vi "Variant to config data - Read.vi"(7 "Section Name":string, 8 "error in (no error)":errorcluster, 9 "Control in":refnum<vi>, 10 "Key Name":string, 11 "FIle refnum IN":T1) -> (0 "error out":errorcluster, 2 "Value":variant, 3 "Refnum out":T1)   [LabVIEW 2017]
uses:
  <vilib>/Utility/config.llb/Config Data RefNum.ctl
  <vilib>/Utility/config.llb/Read Key (String).vi
  <vilib>/Utility/config.llb/Read Key (Double).vi
  <vilib>/Utility/config.llb/Read Key (Boolean).vi
  <vilib>/Utility/config.llb/Read Key (I32).vi
  <vilib>/Utility/config.llb/Read Key (U32).vi
  <vilib>/Utility/config.llb/NI_LVConfig.lvlib
  <vilib>/Utility/Data Type/NI_Data Type.lvlib
panel:
  out "found?":bool
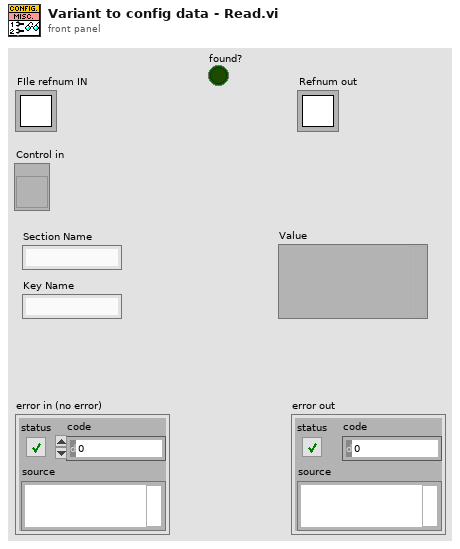
[diagram p1: front panel]
types:
  T1 = typedef "NI_LVConfig.lvlib/Config Data RefNum.ctl" = refnum<k1>
  T2 = typedef "NI_Data Type.lvlib/Data Type.ctl" = enum8{"Invalid Type", "Void", "I8", "I16", "I32", "I64", "U8", "U16", "U32", "U64", "Single Float", "Double Float", "Extended Float", "Single Complex", "Double Complex", "Extended Complex", "Enum U8", "Enum U16", "Enum U32", "Enum U64", "Single Float With Unit", "Double Float With Unit", "Extended Float With Unit", "Single Complex with Unit", "Double Complex with Unit", "Extended Complex with Unit", "Boolean", "String", "Path", "Picture", "Tag", "Array", "Cluster", "Variant", "LV Variant", "Waveform", "Timestamp", "Digital Waveform", "Digital Data", "ExpressData", "Refnum", "External Data", "VI", "Poly VI", "LabVIEW Class Instance", "Fixed Point"}
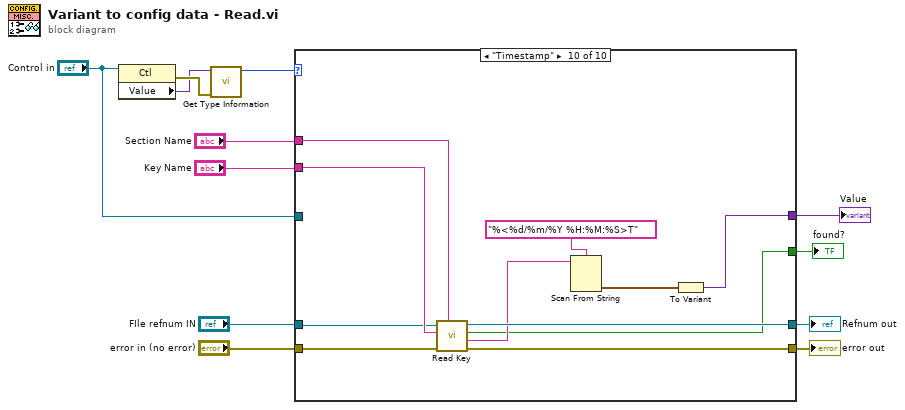
[diagram p0: block diagram]
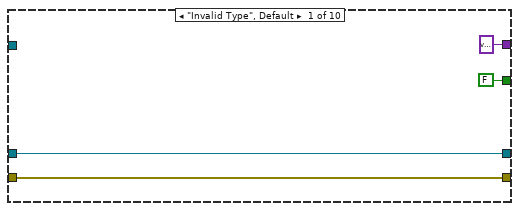
[diagram p2: hidden frame]
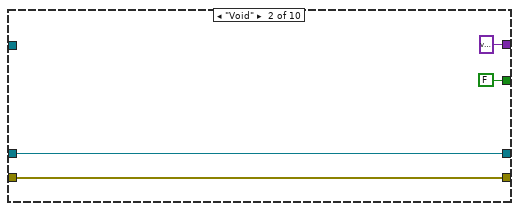
[diagram p3: hidden frame]
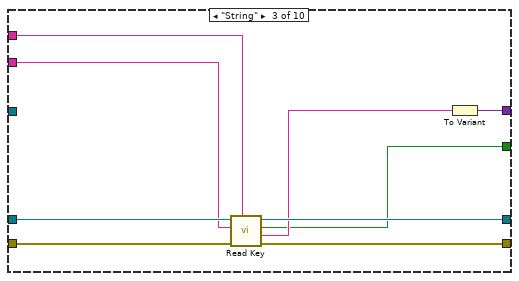
[diagram p4: hidden frame]
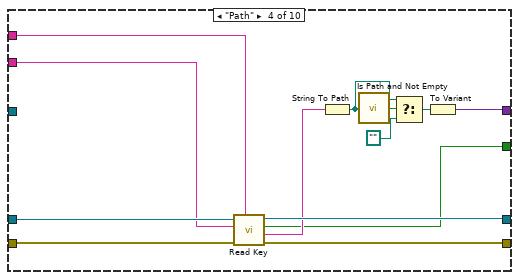
[diagram p5: hidden frame]
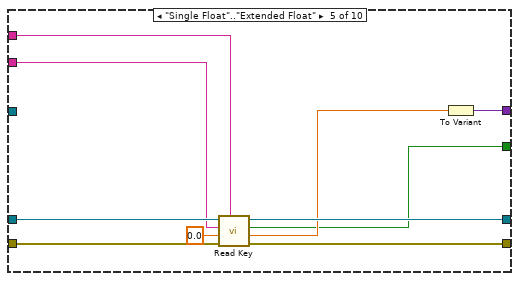
[diagram p6: hidden frame]
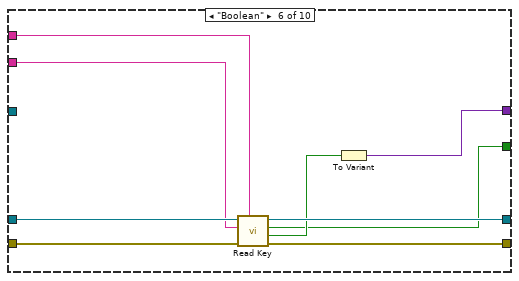
[diagram p7: hidden frame]
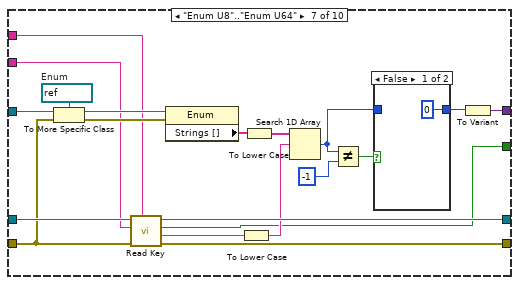
[diagram p8: hidden frame]
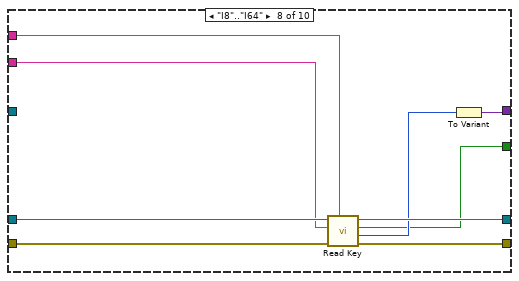
[diagram p10: hidden frame]
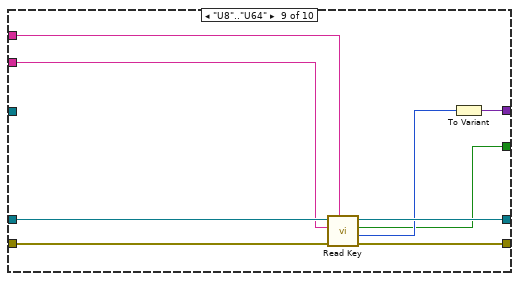
[diagram p11: hidden frame]
diagram:
  n1 = property class="Ctl"(reference="Control in") -> (error out=w5:errorcluster, "Value"=w4:variant)  [unwired: 1 in, 1 out]
  n2 = call <vilib>:"Get Type Information.vi"("error in (no error)"=w5, "Variant"=w4) -> ("Type"=w3:T2)  [unwired: 5 in, 4 out]
  n3 = case shown="\"Timestamp\"" w3 {
    tunnel: "error in (no error)" -> [w15 w19 w29 w42 w51 w60 w76 w91 w100 w109]
    tunnel: "FIle refnum IN" -> [w16 w20 w28 w41 w52 w61 w77 w92 w101 w110]
    tunnel: "Section Name" -> [_ _ w27 w38 w47 w56 w74 w89 w98 w111]
    tunnel: "Key Name" -> [_ _ w26 w37 w48 w57 w73 w90 w99 w112]
    tunnel: [w16 w20 w25 w40 w50 w59 w78 w88 w97 w108] -> w11
    tunnel: [w15 w19 w24 w39 w49 w58 w75 w87 w96 w107] -> w12
    tunnel: [variant ("Variant") variant ("Variant") w22 w35 w45 w55 w64 w86 w95 w103] -> w6
    tunnel: "Control in" -> [_ _ _ _ _ _ w63 _ _ _]
    tunnel: [FALSE ("found?") FALSE ("found?") w21 w30 w43 w53 w62 w84 w93 w102] -> w1
    frame "Invalid Type", Default {
    }
    frame "Void" {
    }
    frame "String" {
      n4 = call-poly <vilib>:"Read Key.vi"("section"=w27, "error in (no error)"=w29, "key"=w26, "refnum"=w28) -> ("error out"=w24:errorcluster, "value"=w23:string, "found?"=w21:bool, "refnum out"=w25:T1)  [unwired: 4 in]
      n5 = To Variant(anything=w23) -> (Variant=w22:variant)
    }
    frame "Path" {
      n6 = call-poly <vilib>:"Read Key.vi"("section"=w38, "error in (no error)"=w42, "key"=w37, "refnum"=w41) -> ("error out"=w39:errorcluster, "value"=w36:string, "found?"=w30:bool, "refnum out"=w40:T1)  [unwired: 4 in]
      n7 = String To Path(string=w36) -> (path=w32:path)
      n8 = call <vilib>:"Is Path and Not Empty.vi"("path"=w32) -> ("Is Path and Not Empty?"=w33:bool)  [unwired: 4 in]
      n9 = Select(t=w32, s=w33, f=path "") -> (s? t:f=w34:path)
      n10 = To Variant(anything=w34) -> (Variant=w35:variant)
    }
    frame "Single Float".."Extended Float" {
      n11 = call-poly <vilib>:"Read Key.vi"("section"=w47, "error in (no error)"=w51, "default value"=0.0, "key"=w48, "refnum"=w52) -> ("error out"=w49:errorcluster, "value"=w44:dbl, "found?"=w43:bool, "refnum out"=w50:T1)  [unwired: 3 in]
      n12 = To Variant(anything=w44) -> (Variant=w45:variant)
    }
    frame "Boolean" {
      n13 = call-poly <vilib>:"Read Key.vi"("section"=w56, "error in (no error)"=w60, "key"=w57, "refnum"=w61) -> ("error out"=w58:errorcluster, "value"=w54:bool, "found?"=w53:bool, "refnum out"=w59:T1)  [unwired: 4 in]
      n14 = To Variant(anything=w54) -> (Variant=w55:variant)
    }
    frame "Enum U8".."Enum U64" {
      w81 = refnum<vi> refnum  # Enum
      n15 = To More Specific Class(target class=w81, reference=w63, error in=w76) -> (specific class reference=w79:refnum<vi>, error out=w80:errorcluster)
      n16 = call-poly <vilib>:"Read Key.vi"("section"=w74, "error in (no error)"=w76, "key"=w73, "refnum"=w77) -> ("error out"=w75:errorcluster, "value"=w70:string, "found?"=w62:bool, "refnum out"=w78:T1)  [unwired: 4 in]
      n17 = property class="Enum"(reference=w79, error in=w80) -> ("Strings []"=w72:string[])  [unwired: 2 out]
      n18 = To Lower Case(string=w70) -> (all lower case string=w69:string)
      n19 = To Lower Case(string=w72) -> (all lower case string=w71:string[])
      n20 = Search 1D Array(1D array=w71, element=w69) -> (index of element=w66:i32)  [unwired: 1 in]
      n21 = Not Equal?(x=w66, y=-1) -> (x != y?=w67:bool)
      n22 = case shown="False" w67 {
        tunnel: w66 -> [_ w83]
        tunnel: [0 ("index of element") w83] -> w65
        frame False {
        }
        frame True {
        }
      }
      n23 = To Variant(anything=w65) -> (Variant=w64:variant)
    }
    frame "I8".."I64" {
      n24 = call-poly <vilib>:"Read Key.vi"("section"=w89, "error in (no error)"=w91, "key"=w90, "refnum"=w92) -> ("error out"=w87:errorcluster, "value"=w85:i32, "found?"=w84:bool, "refnum out"=w88:T1)  [unwired: 4 in]
      n25 = To Variant(anything=w85) -> (Variant=w86:variant)
    }
    frame "U8".."U64" {
      n26 = call-poly <vilib>:"Read Key.vi"("section"=w98, "error in (no error)"=w100, "key"=w99, "refnum"=w101) -> ("error out"=w96:errorcluster, "value"=w94:u32, "found?"=w93:bool, "refnum out"=w97:T1)  [unwired: 4 in]
      n27 = To Variant(anything=w94) -> (Variant=w95:variant)
    }
    frame "Timestamp" {
      n28 = call-poly <vilib>:"Read Key.vi"("section"=w111, "error in (no error)"=w109, "key"=w112, "refnum"=w110) -> ("error out"=w107:errorcluster, "value"=w105:string, "found?"=w102:bool, "refnum out"=w108:T1)  [unwired: 4 in]
      n29 = Scan From String(format string="%<%d/%m/%Y %H:%M:%S>T", input string=w105) -> (output 1=w104:timestamp)  [unwired: 3 in, 3 out]
      n30 = To Variant(anything=w104) -> (Variant=w103:variant)
    }
  }
  "error out" <- w12
  "Refnum out" <- w11
  "Value" <- w6
  "found?" <- w1
